vi "MGI Smoothed Interpolation Weights.vi"(2 "x":dbl, 3 "x Array[]":dbl[](array[numeric])) -> (0 "Weights[]":dbl[](array[numeric]), 1 "Indices":i32[](array[numeric]))   [LabVIEW 2020]
doc: "Calculate the weights needed for a smoothed interpolation of an irregularly sampled function. Linear fit is made through endpoints, then cosine functions handle deviations from linearity.\n\ny=mx + (yA + yB - m(xA + xB))/2 - (yB - yA - m(xB - xA))(cos(pi(x - xA)/(xB - xA))/2\n\nUnlike a spline fit, weights can be precalculated and applied for any y values.\n\n\nAuthored by David A. Moore\nsupport@mooregoodideas.com\nwww.mooregoodideas.com\n\nCopyright (c) 2010, Moore Good Ideas, Inc.\n\nAll rights reserved.\n\nRedistribution and use in source and binary forms, with or without modification, are permitted provided that the following conditions are met:\n\n * Redistributions of source code must retain the above copyright notice, this list of conditions and the following disclaimer.\n * Redistributions in binary form must reproduce the above copyright notice, this list of conditions and the following disclaimer in the documentation and/or other materials provided with the distribution.\n * Neither the name of Moore Good Ideas, Inc. nor the names of its contributors may be used to endorse or promote products derived from this software without specific prior written permission.\n\nTHIS SOFTWARE IS PROVIDED BY THE COPYRIGHT HOLDERS AND CONTRIBUTORS \"AS IS\" AND ANY EXPRESS OR IMPLIED WARRANTIES, INCLUDING, BUT NOT LIMITED TO, THE IMPLIED WARRANTIES OF MERCHANTABILITY AND FITNESS FOR A PARTICULAR PURPOSE ARE DISCLAIMED. IN NO EVENT SHALL THE COPYRIGHT OWNER OR CONTRIBUTORS BE LIABLE FOR ANY DIRECT, INDIRECT, INCIDENTAL, SPECIAL, EXEMPLARY, OR CONSEQUENTIAL DAMAGES (INCLUDING, BUT NOT LIMITED TO, PROCUREMENT OF SUBSTITUTE GOODS OR SERVICES; LOSS OF USE, DATA, OR PROFITS; OR BUSINESS INTERRUPTION) HOWEVER CAUSED AND ON ANY THEORY OF LIABILITY, WHETHER IN CONTRACT, STRICT LIABILITY, OR TORT (INCLUDING NEGLIGENCE OR OTHERWISE) ARISING IN ANY WAY OUT OF THE USE OF THIS SOFTWARE, EVEN IF ADVISED OF THE POSSIBILITY OF SUCH DAMAGE."
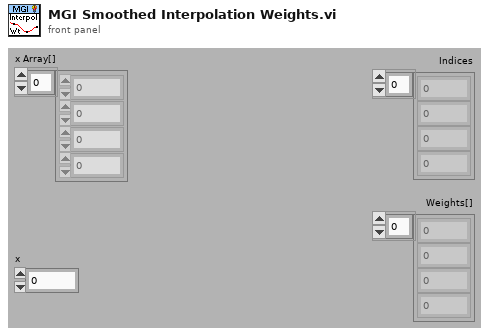
[diagram p1: front panel]
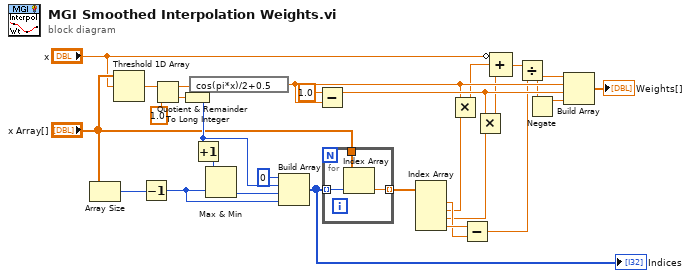
[diagram p0: block diagram]
diagram:
  n1 = Array Size(array="x Array[]") -> (size(s)=w23:i32)
  n2 = Threshold 1D Array(2:"x", 3:"x Array[]") -> (0:w28:dbl)  [unwired: 1 out]
  n3 = Decrement(x=w23) -> (x-1=w21:i32)
  n4 = Quotient & Remainder(x=w28, y=1.0) -> (x-y*floor(x/y)=w25:dbl, floor(x/y)=w26:dbl)
  n5 = To Long Integer(number=w26) -> (32bit integer=w20:i32)
  n6 = expression code="cos(pi*x)/2+0.5"(w25) -> (w9:dbl)
  n7 = Increment(x=w20) -> (x+1=w24:i32)
  n8 = Max & Min(x=w24, y=w21) -> (min(x,y)=w22:i32)  [unwired: 1 out]
  n9 = Build Array(0 ("element"), w20, w22, w21) -> (w17:i32[])
  "Indices" <- w17
  n10 = Subtract(x=1.0, y=w9) -> (x-y=w11:dbl)
  n11 = for {
    tunnel: "x Array[]" -> [w31]
    tunnel: w17 -> [w30] mode=indexing
    tunnel: [w29] -> w16 mode=indexing
    n12 = Index Array(array=w31, index=w30) -> (element=w29:dbl)
  }
  n13 = Index Array(array=w16) -> (element #1=w13:dbl, element #2=w10:dbl, element #3=w12:dbl, element #4=w14:dbl)  [unwired: 4 in]
  n14 = Multiply(x=w9, y=w10) -> (x*y=w8:dbl)
  n15 = Subtract(x=w14, y=w13) -> (x-y=w4:dbl)
  n16 = Multiply(x=w11, y=w12) -> (x*y=w7:dbl)
  n17 = Compound Arithmetic op=ADD(invert "x", w8, w7) -> (w5:dbl)
  n18 = Divide(x=w5, y=w4) -> (x/y=w3:dbl)
  n19 = Negate(x=w3) -> (-x=w2:dbl)
  n20 = Build Array(w3, w9, w11, w2) -> (→"Weights[]":dbl[])
